vi "Close Form.vi"(8 "error in (no error)":errorcluster, 10 "Form Name":T1, 11 "Form Server in":refnum<class "Form Server.lvclass">) -> (0 "error out":errorcluster, 3 "Form Server out":refnum<class "Form Server.lvclass">)   [LabVIEW 2020, in "Form Server.lvlib" / "Form Server.lvclass"]
uses:
  Form Server.lvclass
  Autoclose manager/Form ID.ctl
  Form Server.lvclass/Form Server.ctl
  Form Server Interfaces.lvlib
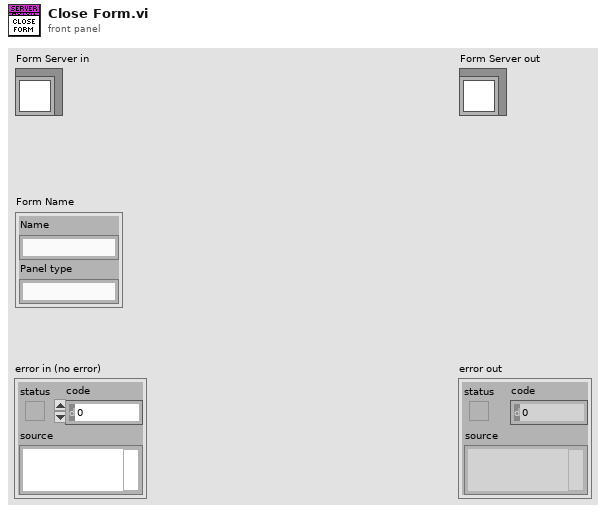
[diagram p1: front panel]
types:
  T1 = typedef "Form Server Interfaces.lvlib/Form ID.ctl" = cluster{"Name":string, "Panel type":string}
  T2 = map{T1, refnum<class "Message Enqueuer.lvclass">}
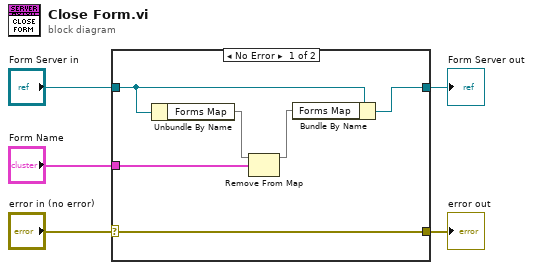
[diagram p0: block diagram]
diagram:
  n1 = case shown="No Error" "error in (no error)" {
    selector: "error in (no error)" -> [w7 w13]
    tunnel: [w7 w13] -> w4
    tunnel: [w9 w12] -> w2
    tunnel: "Form Server in" -> [w10 w12]
    tunnel: "Form Name" -> [w6 _]
    frame No Error {
      n2 = Unbundle By Name(w10) -> ("Forms Map"=w11:T2)
      n3 = Remove From Map(10:w6, 11:w11) -> (3:w8:T2)  [unwired: 2 out]
      n4 = Bundle By Name(cluster=w10, "Forms Map"=w8) -> (w9:refnum<class "Form Server.lvclass">)
    }
    frame Error {
    }
  }
  "error out" <- w4
  "Form Server out" <- w2
